vi "main_real-time HMI for air-wrting to input characters 23.3.3.vi"() -> ()   [LabVIEW 2020]
uses:
  <vilib>/Analysis/3filter.llb/Filter Passband Type.ctl
  <vilib>/Analysis/NI_AALBase.lvlib
  <vilib>/Analysis/3filter.llb/Butterworth Filter (DBL).vi
  <vilib>/express/express analysis/Spectral/XNode/ExpressSpectralMeasurementsBlockNode.xnode
  <vilib>/express/express analysis/Spectral/Block/exnSpectralBlock spectral measurements power poly.vi
  <vilib>/Analysis/NI_AALPro.lvlib
  <vilib>/Analysis/NI_AAL_SigProc.lvlib
  <vilib>/Utility/file.llb/Write Delimited Spreadsheet (DBL).vi
  <vilib>/express/express analysis/Spectral/Block/exnSpectralBlock spectral measurements power DDT.vi
panel:
  out "最大值 2":dbl
  out "手势":dbl
  in  "训练——手势":string
  out "卡尔曼滤波":cluster{"Y":dbl[], "Y":dbl[]}[](graph)
  out "通道1":dynamicdata(graph)
  out "XY Graph 2":cluster{"Y":dbl[], "Y":dbl[]}[](graph) caption="ML_集成树"
  in  "训练——位置":dbl
  out "数值":dbl
  out "采样点 2":dbl
  out "采样点":dbl
  out "ToF 2(cm)":dbl
  out "ToF 1(cm)":dbl
  out "有手势":bool
  out "最大值 1":dbl
  out "最大值2":dbl
  out "波形图 2":dbl[](graph)
  out "余数 2":dbl
  out "循环 2":dbl
  out "波形图":dbl[](graph)
  out "通道1_去环境噪声":dbl[](graph)
  out "通道2_去环境+滤波":dbl[](graph)
  out "频谱2":dynamicdata(graph)
  out "通道1_滤波":dbl[](graph)
  out "通道2_滤波":dbl[](graph)
  out "激励信号":dynamicdata(graph)
  out "通道2":dynamicdata(graph)
  in  "停止":bool
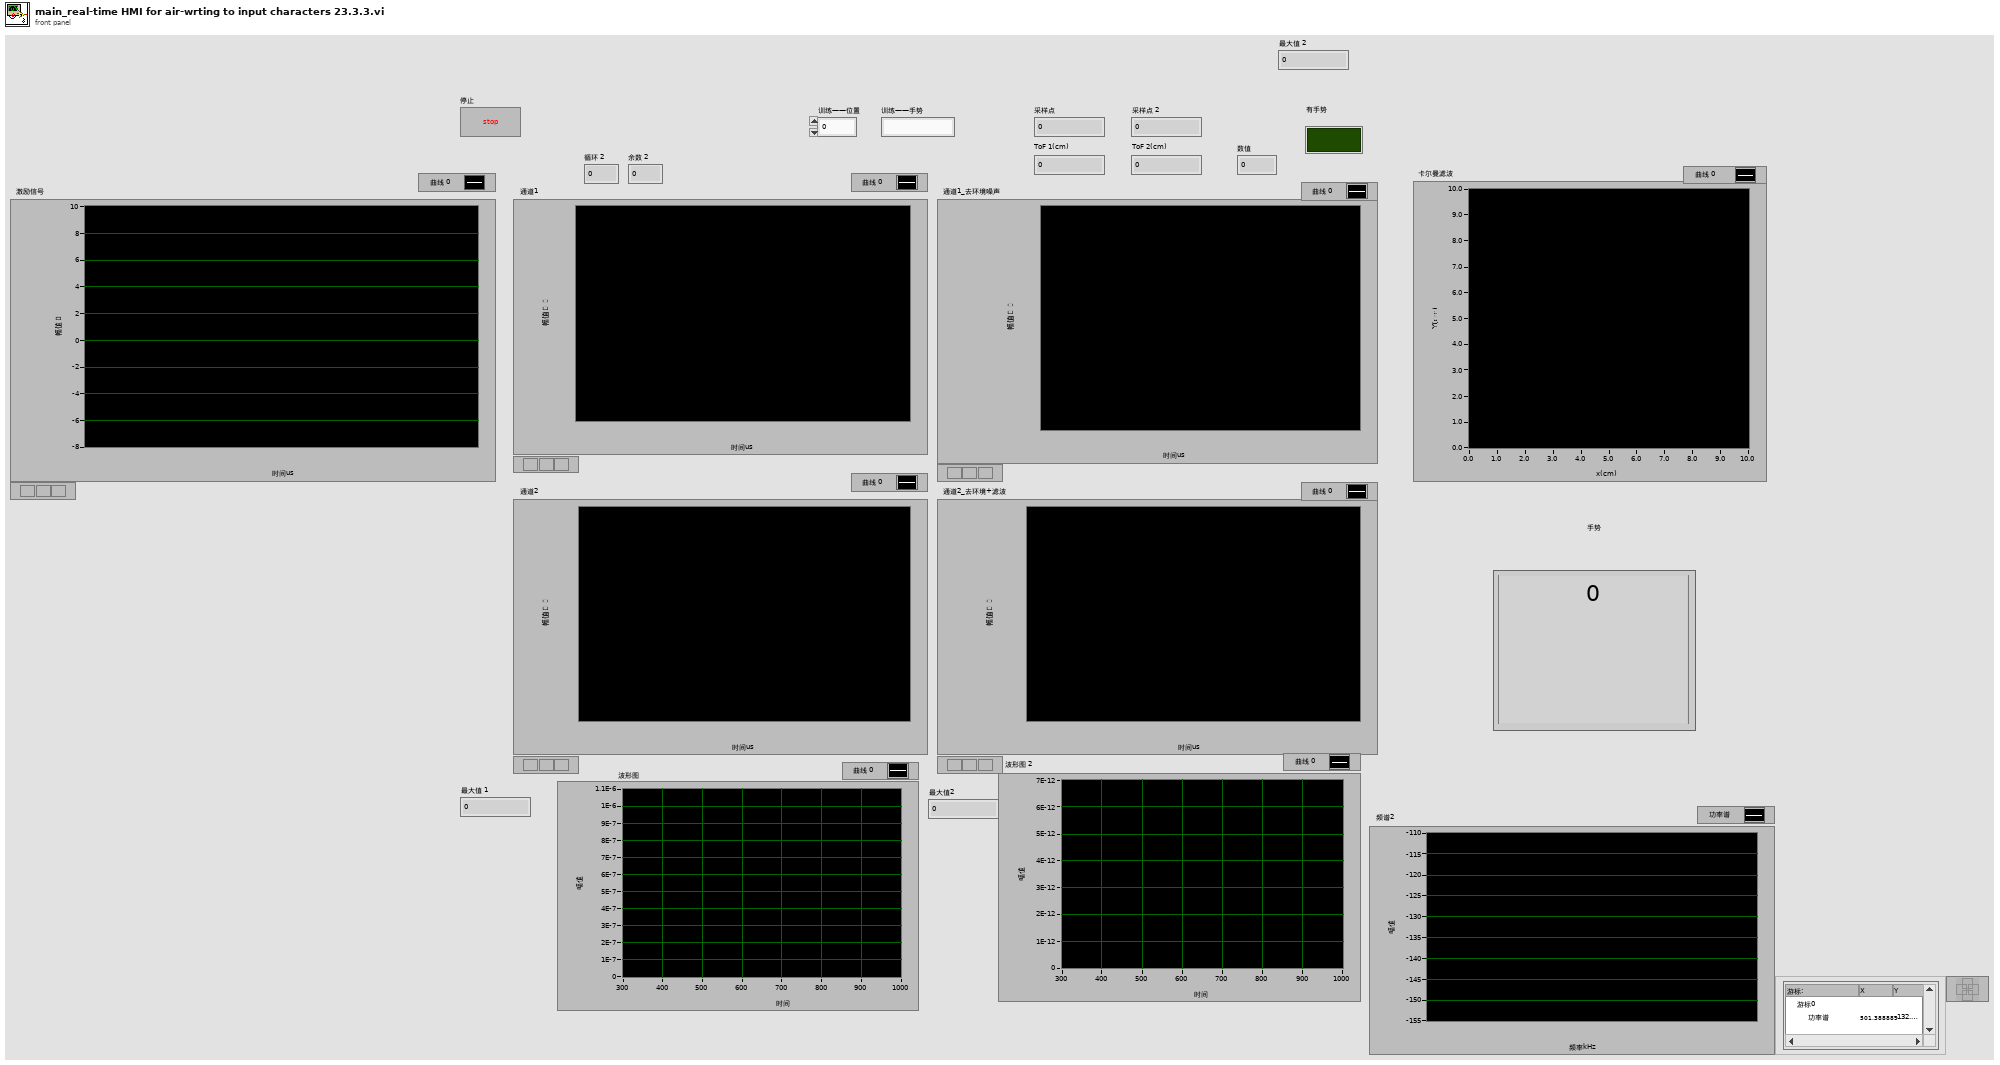
[diagram p1: front panel]
types:
  T1 = typedef "NI_AALBase.lvlib/Filter Passband Type.ctl" = enum32{"Lowpass", "Highpass", "Bandpass", "Bandstop"}
  T2 = cluster{"averaging mode":u16, "weighting mode":u16, "number of averages":u32}
  T3 = cluster{"dB On (F)":bool, "unwrap phase (F)":bool, "convert to degree (F)":bool}
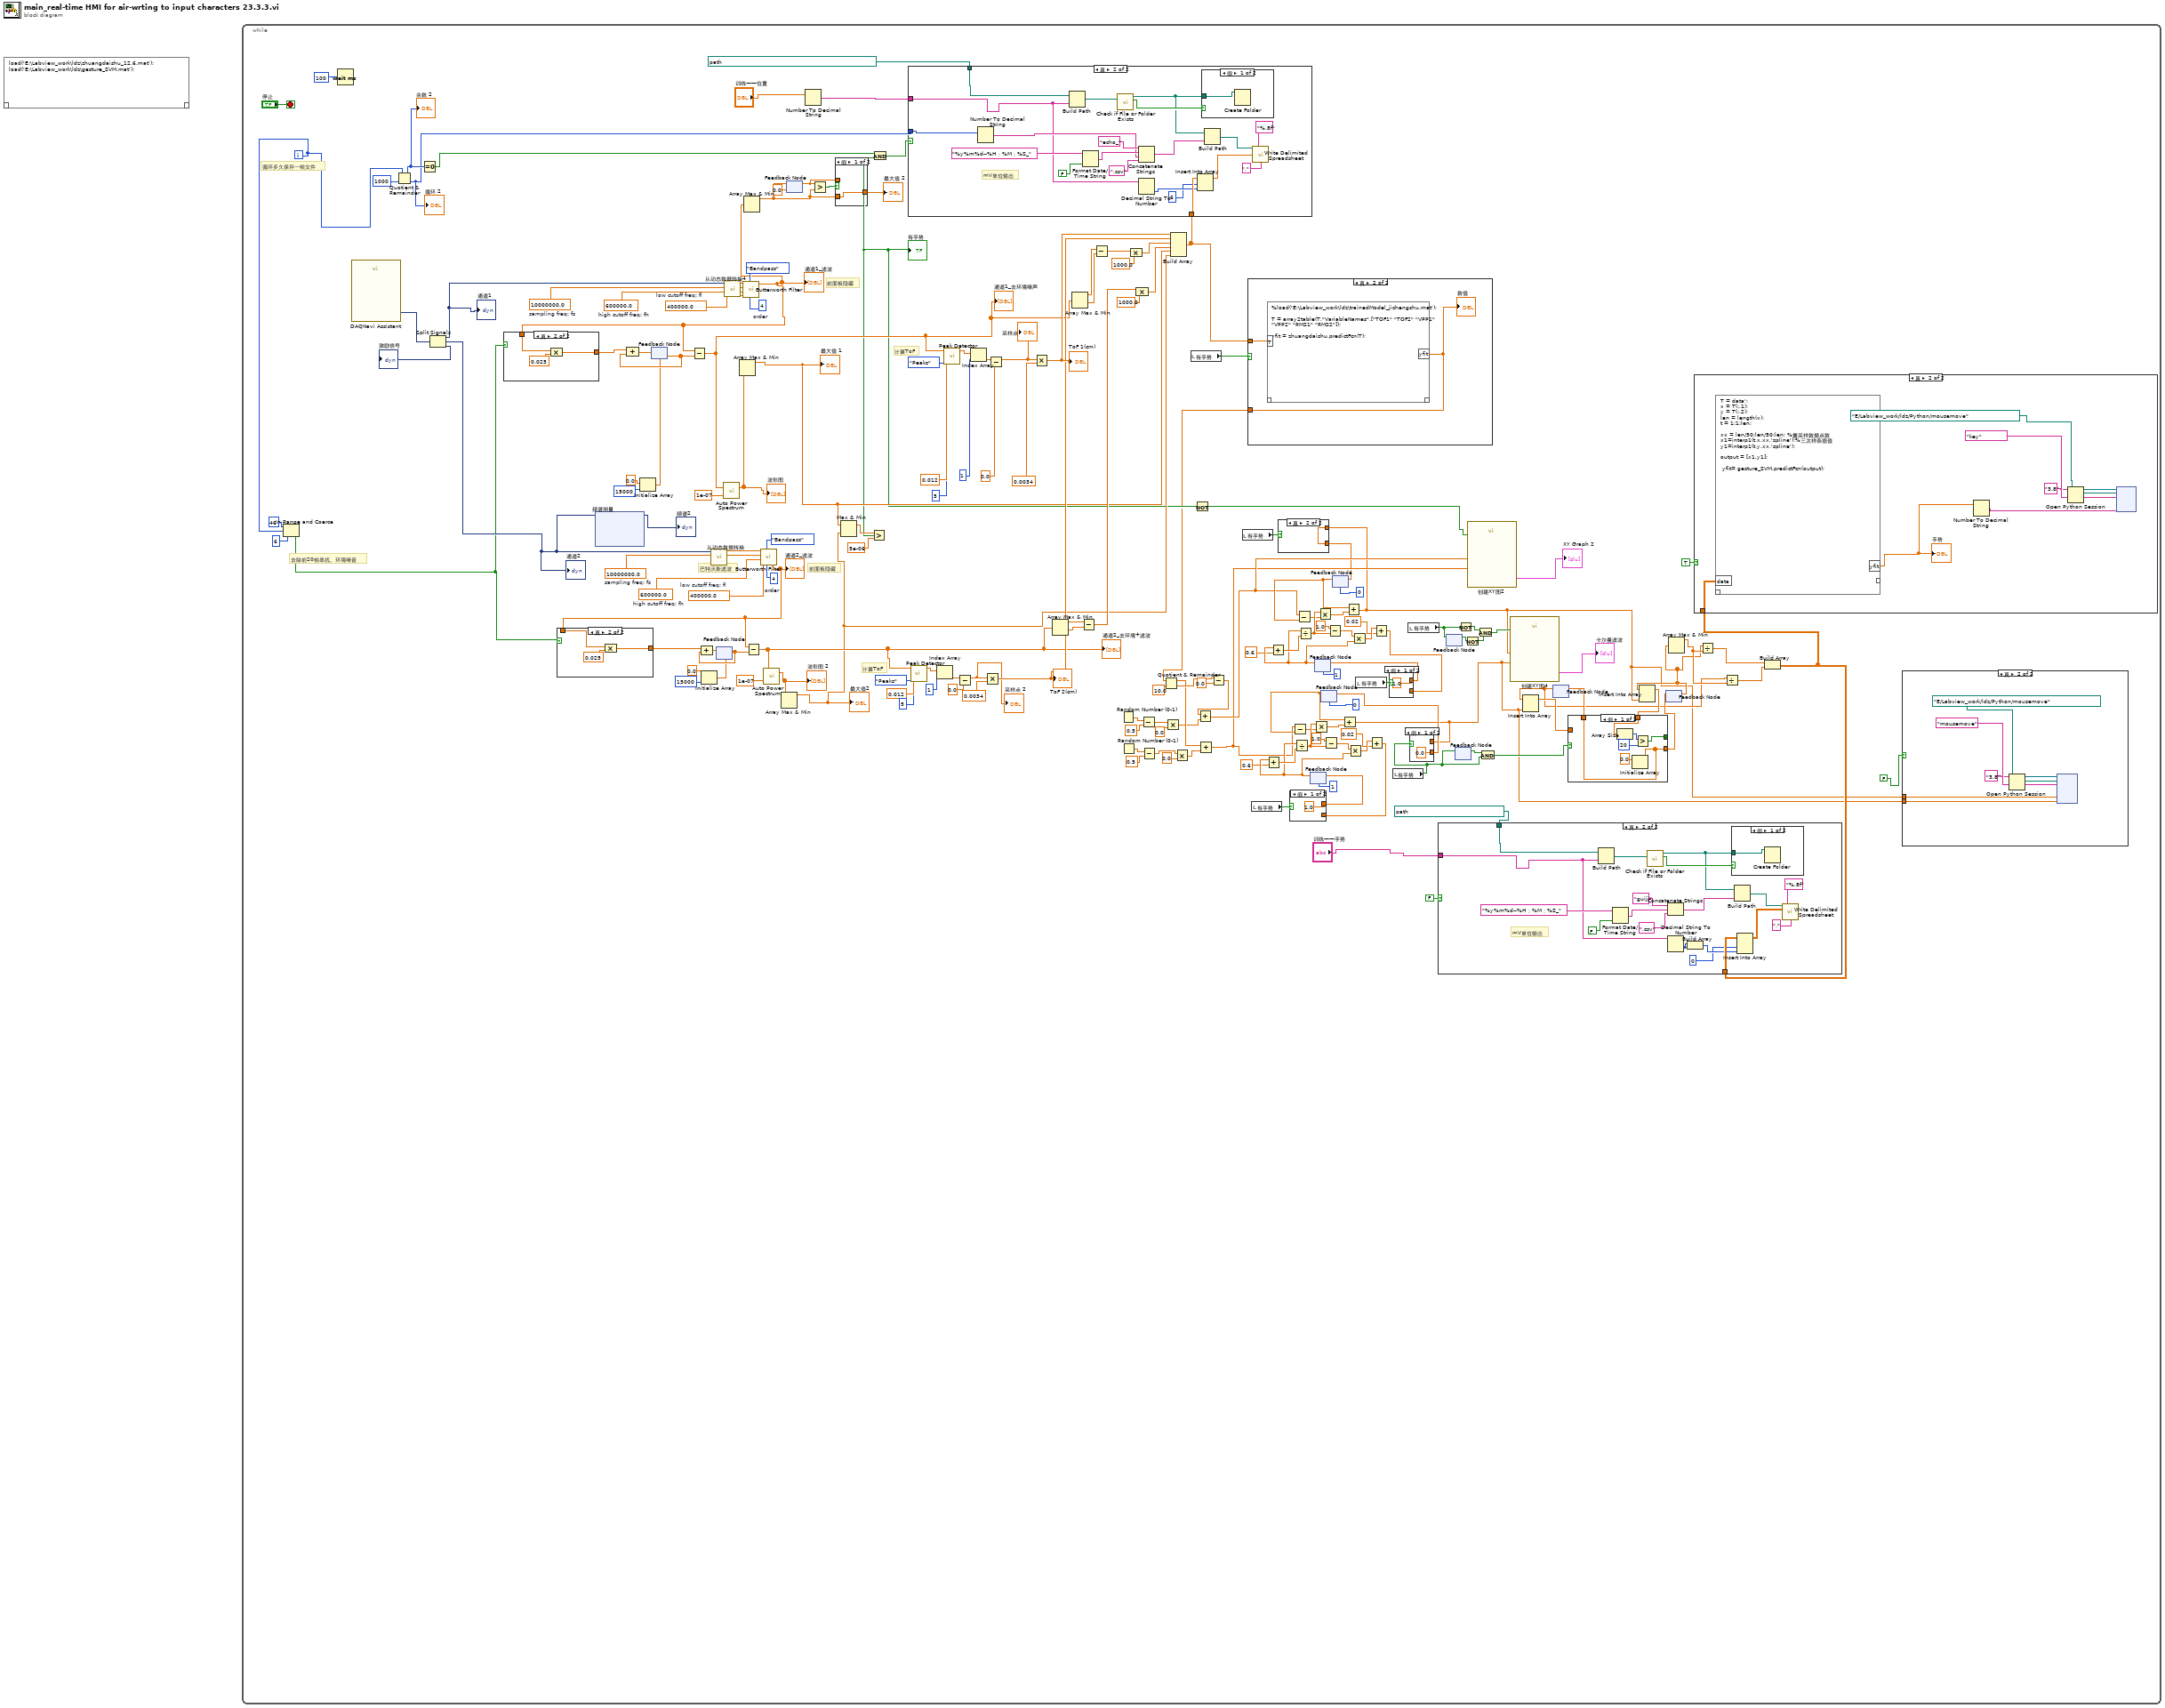
[diagram p0: block diagram]
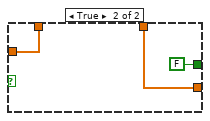
[diagram p7: hidden frame]
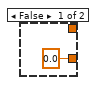
[diagram p11: hidden frame]
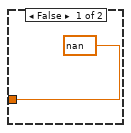
[diagram p12: hidden frame]
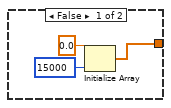
[diagram p15: hidden frame]
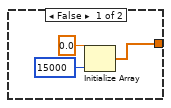
[diagram p16: hidden frame]
diagram:
  n1 = script code="load('E:\\Labview_work\\ldz\\zhuangdaishu_12.6.mat');\nload('E:\\Labview_work\\ldz\\gesture_SVM.mat');"() -> ()  [unwired: 1 in, 1 out]
  n2 = while {
    i -> [w139]
    stop <- "停止" stop-if-true
    w161 = 400000.0  # low cutoff freq: fl
    w165 = 600000.0  # high cutoff freq: fh
    w164 = 10000000.0  # sampling freq: fs
    w166 = 4  # order
    w172 = 400000.0  # low cutoff freq: fl
    w171 = 600000.0  # high cutoff freq: fh
    w170 = 10000000.0  # sampling freq: fs
    w173 = 4  # order
    # "计算ToF"
    # "计算ToF"
    # "前面板隐藏"
    # "前面板隐藏"
    # "去除前20帧串扰、环境噪音"
    # "循环多久保存一帧文件"
    # "巴特沃斯滤波"
    n3 = In Range and Coerce(upper limit=46 ("上限"), x=w139, lower limit=6 ("下限")) -> (In Range?=w143:bool)  [unwired: 1 out]
    n4 = Wait (ms)(milliseconds to wait=100) -> ()  [unwired: 1 out]
    n5 = call "DAQNavi Assistant"() -> ("data out(DDT)"=w159:dynamicdata)  [unwired: 6 in, 21 out]
    n6 = Quotient & Remainder(x=w139, y=1000) -> (x-y*floor(x/y)=w141:i32, floor(x/y)=w140:i32)
    "循环 2" <- w140
    "余数 2" <- w141
    n7 = Equal To 0?(x=w141) -> (x = 0?=w130:bool)
    n8 = Split Signals(w159) -> (w93:dynamicdata, w160:dynamicdata, →"激励信号":dynamicdata)  [unwired: 3 in]
    "通道2" <- w160
    "通道1" <- w93
    n9 = xnode "频谱测量"("信号"=w160) -> ("功率谱"=→"频谱2":dynamicdata)  [unwired: 1 in, 1 out]
    n10 = Initialize Array(0.0 ("元素"), 15000 ("维数大小")) -> (w147:dbl[])
    n11 = feedback #1(w147) -> (w149:dbl[])
    n12 = Initialize Array(0.0 ("元素"), 15000 ("维数大小")) -> (w155:dbl[])
    n13 = call "从动态数据转换"("Dynamic Data Type"=w160) -> ("Array"=w168:dbl[])  [unwired: 3 in]
    n14 = feedback #2(w155) -> (w156:dbl[])
    n15 = call "从动态数据转换4"("Dynamic Data Type"=w93) -> ("Array"=w162:dbl[])  [unwired: 3 in]
    n16 = call-poly <vilib>:"Butterworth Filter.vi"("order"=w166, "filter type"=Filter_Passband_Type."Bandpass", "low cutoff freq: fl"=w161, "high cutoff freq: fh"=w165, "sampling freq: fs"=w164, "X"=w162) -> ("Filtered X"=w6:dbl[])  [unwired: 2 in, 1 out]
    "通道1_滤波" <- w6
    n17 = case shown="真" w143 {
      tunnel: w6 -> [_ w254]
      tunnel: [w251 w256] -> w151
      frame False {
        n18 = Initialize Array(0.0 ("元素"), 15000 ("维数大小")) -> (w251:dbl[])
      }
      frame True {
        n19 = Compound Arithmetic op=MULTIPLY(w254, 0.025) -> (w256:dbl[])
      }
    }
    n20 = Compound Arithmetic op=ADD(w151, w149) -> (w150:dbl[])
    n21 = feedback-in #1(w150) -> ()
    n22 = Subtract(x=w6, y=w149) -> (x-y=w109:dbl[])
    "通道1_去环境噪声" <- w109
    n23 = call <vilib>:"Auto Power Spectrum.vi"("dt"=1e-07, "Signal (V)"=w109) -> ("Power Spectrum (V^2 rms)"=w133:dbl[])  [unwired: 1 out]
    "波形图" <- w133
    n24 = Array Max & Min(array=w133) -> (max value=w100:dbl)  [unwired: 3 out]
    "最大值 1" <- w100
    n25 = Array Max & Min(array=w6) -> (max value=w3:dbl)  [unwired: 3 out]
    n26 = call-poly <vilib>:"Butterworth Filter.vi"("order"=w173, "filter type"=Filter_Passband_Type."Bandpass", "low cutoff freq: fl"=w172, "high cutoff freq: fh"=w171, "sampling freq: fs"=w170, "X"=w168) -> ("Filtered X"=w152:dbl[])  [unwired: 2 in, 1 out]
    "通道2_滤波" <- w152
    n27 = case shown="真" w143 {
      tunnel: w152 -> [_ w262]
      tunnel: [w257 w261] -> w158
      frame False {
        n28 = Initialize Array(0.0 ("元素"), 15000 ("维数大小")) -> (w257:dbl[])
      }
      frame True {
        n29 = Compound Arithmetic op=MULTIPLY(w262, 0.025) -> (w261:dbl[])
      }
    }
    n30 = Compound Arithmetic op=ADD(w158, w156) -> (w157:dbl[])
    n31 = feedback-in #2(w157) -> ()
    n32 = Subtract(x=w152, y=w156) -> (x-y=w108:dbl[])
    "通道2_去环境+滤波" <- w108
    n33 = call <vilib>:"Auto Power Spectrum.vi"("dt"=1e-07, "Signal (V)"=w108) -> ("Power Spectrum (V^2 rms)"=w134:dbl[])  [unwired: 1 out]
    "波形图 2" <- w134
    n34 = Array Max & Min(array=w134) -> (max value=w99:dbl)  [unwired: 3 out]
    "最大值2" <- w99
    n35 = feedback #3(0.0) -> (w2:dbl)
    n36 = feedback-in #3(w3) -> ()
    n37 = Number To Decimal String(number="训练——位置") -> (decimal integer string=w95:string)  [unwired: 1 in]
    n38 = Greater?(x=w2, y=w3) -> (0:w4:bool)
    n39 = case shown="假" w4 {
      tunnel: w3 -> [w175 _]
      tunnel: w2 -> [_ w176]
      tunnel: [w175 w176] -> w1
      frame False {
      }
      frame True {
      }
    }
    "最大值 2" <- w1
    n40 = Max & Min(x=w100, y=w99) -> (max(x,y)=w132:dbl)  [unwired: 1 out]
    n41 = Greater?(x=w132, y=5e-06) -> (0:w98:bool)
    "有手势" <- w98
    n42 = And(x=w130, y=w98) -> (x .and. y?=w129:bool)
    n43 = call <vilib>:"Peak Detector.vi"("peaks/valleys"=enum32{"Peaks", "Valleys"}."Peaks", "width"=5, "threshold"=0.012, "X"=w108) -> ("Locations"=w120:dbl[])  [unwired: 3 in, 4 out]
    n44 = Index Array(array=w120, index=1 ("索引")) -> (element=w89:dbl)
    n45 = call <vilib>:"Peak Detector.vi"("peaks/valleys"=enum32{"Peaks", "Valleys"}."Peaks", "width"=5, "threshold"=0.012, "X"=w109) -> ("Locations"=w125:dbl[])  [unwired: 3 in, 4 out]
    n46 = Subtract(x=w89, y=0.0) -> (x-y=w90:dbl)
    "采样点 2" <- w90
    n47 = Index Array(array=w125, index=1 ("索引")) -> (element=w118:dbl)
    n48 = Multiply(x=w90, y=0.0034) -> (x*y=w113:dbl)
    "ToF 2(cm)" <- w113
    n49 = Subtract(x=w118, y=0.0) -> (x-y=w92:dbl)
    "采样点" <- w92
    n50 = Multiply(x=w92, y=0.0034) -> (x*y=w114:dbl)
    "ToF 1(cm)" <- w114
    n51 = Array Max & Min(array=w108) -> (max value=w103:dbl, min value=w102:dbl)  [unwired: 2 out]
    n52 = Array Max & Min(array=w109) -> (max value=w107:dbl, min value=w106:dbl)  [unwired: 2 out]
    n53 = Subtract(x=w103, y=w102) -> (x-y=w104:dbl)
    n54 = Subtract(x=w107, y=w106) -> (x-y=w105:dbl)
    n55 = Random Number (0-1)() -> (number: 0 to 1=w84:dbl)
    n56 = Random Number (0-1)() -> (number: 0 to 1=w81:dbl)
    n57 = Compound Arithmetic op=MULTIPLY(w105, 1000.0) -> (w111:dbl)
    n58 = Compound Arithmetic op=MULTIPLY(w104, 1000.0) -> (w101:dbl)
    n59 = Subtract(x=w84, y=0.5) -> (x-y=w78:dbl)
    n60 = Subtract(x=w81, y=0.5) -> (x-y=w73:dbl)
    n61 = Multiply(x=w78, y=0.0) -> (x*y=w77:dbl)
    n62 = Build Array(w114, w113, w111, w101, w100, w99) -> (w97:dbl[])
    n63 = case shown="真" w129 {
      tunnel: w140 -> [_ w240]
      tunnel: path "E:/Labview_work/ldz/数据/3.3/test" ("路径") -> [_ w237]
      tunnel: w97 -> [_ w235]
      tunnel: w95 -> [_ w230]
      frame False {
      }
      frame True {
        # "mV单位输出"
        n64 = Number To Decimal String(number=w240) -> (decimal integer string=w239:string)  [unwired: 1 in]
        n65 = Build Path(base path=w237, name or relative path=w230) -> (appended path=w244:path)
        n66 = Format Date/Time String ("格式化日期/时间字符串")(time format string (%c)="%y%m%d--%H：%M：%S_", UTC format=FALSE) -> (date/time string=w246:string)  [unwired: 1 in]
        n67 = call <vilib>:"Check if File or Folder Exists.vi"("path"=w244) -> ("file or folder exists?"=w243:bool, "dup path"=w231:path)  [unwired: 8 in, 1 out]
        n68 = Concatenate Strings("echo_" ("字符串"), w246, w239, ".csv" ("字符串")) -> (w248:string)
        n69 = Decimal String To Number(string=w230) -> (number=w233:i32)  [unwired: 2 in, 1 out]
        n70 = Insert Into Array(array=w235, index=6 ("索引"), new element=w233) -> (w234:dbl[])
        n71 = case shown="假" w243 {
          tunnel: w231 -> [w250 _]
          frame False {
            n72 = Create Folder(path (use dialog)=w250) -> ()  [unwired: 2 in, 3 out]
          }
          frame True {
          }
        }
        n73 = Build Path(base path=w231, name or relative path=w248) -> (appended path=w247:path)
        n74 = call-poly <vilib>:"Write Delimited Spreadsheet.vi"("file path (dialog if empty)"=w247, "format (%.3f)"="%.8f", "1D data"=w234, "delimiter (\\t)"="," ("delimiter (\\t)")) -> ()  [unwired: 10 in, 2 out]
      }
    }
    n75 = Multiply(x=w73, y=0.0) -> (x*y=w74:dbl)
    n76 = local read "有手势"() -> (w43:bool)
    n77 = Not(x=w98) -> (.not. x?=w28:bool)
    n78 = local read "有手势"() -> (w38:bool)
    n79 = case shown="真" w43 {
      tunnel: w97 -> [_ w229]
      tunnel: [nan w228] -> w46
      frame False {
      }
      frame True {
        n80 = script code="%load('E:\\Labview_work\\ldz\\trainedModel_jichengshu.mat');\n\nT = array2table(T,\"VariableNames\",[\"TOF1\" \"TOF2\" \"VPP1\" \"VPP2\" \"RMS1\" \"RMS2\"]);\n\nyfit = zhuangdaishu.predictFcn(T);" ("脚本节点")("T"=w229) -> ("yfit"=w228:dbl)  [unwired: 1 in, 1 out]
        "数值" <- w228
      }
    }
    n81 = Quotient & Remainder(x=w46, y=10.0) -> (x-y*floor(x/y)=w79:dbl, floor(x/y)=w86:dbl)
    n82 = Add(x=w79, y=w74) -> (x+y=w44:dbl)
    n83 = Subtract(x=w86, y=0.0) -> (x-y=w82:dbl)
    n84 = Add(x=w82, y=w77) -> (x+y=w45:dbl)
    n85 = local read "有手势"() -> (w36:bool)
    n86 = feedback #4(1) -> (w52:dbl)
    n87 = Add(x=w52, y=0.6) -> (x+y=w59:dbl)
    n88 = Divide(x=w52, y=w59) -> (x/y=w57:dbl)
    n89 = feedback #5(1) -> (w65:dbl)
    n90 = Add(x=w65, y=0.6) -> (x+y=w72:dbl)
    n91 = Divide(x=w65, y=w72) -> (x/y=w70:dbl)
    n92 = feedback #6(0) -> (w51:dbl)
    n93 = Subtract(x=w44, y=w51) -> (x-y=w56:dbl)
    n94 = Multiply(x=w57, y=w56) -> (x*y=w55:dbl)
    n95 = Subtract(x=1.0, y=w57) -> (x-y=w54:dbl)
    n96 = Subtract(x=1.0, y=w70) -> (x-y=w67:dbl)
    n97 = feedback #7(0) -> (w64:dbl)
    n98 = Subtract(x=w45, y=w64) -> (x-y=w69:dbl)
    n99 = Multiply(x=w70, y=w69) -> (x*y=w68:dbl)
    n100 = Add(x=w51, y=w55) -> (x+y=w11:dbl)
    n101 = Add(x=w64, y=w68) -> (x+y=w12:dbl)
    n102 = case shown="真" w38 {
      tunnel: w12 -> [_ w226]
      tunnel: [0.0 w226] -> w37
      frame False {
      }
      frame True {
      }
    }
    n103 = feedback-in #7(w37) -> ()
    n104 = Multiply(x=w54, y=w52) -> (x*y=w53:dbl)
    n105 = Multiply(x=w67, y=w65) -> (x*y=w66:dbl)
    n106 = local read "有手势"() -> (w31:bool)
    n107 = Add(x=w53, y=0.02) -> (x+y=w35:dbl)
    n108 = case shown="假" w36 {
      tunnel: w35 -> [_ w224]
      tunnel: [1.0 w224] -> w34
      frame False {
      }
      frame True {
      }
    }
    n109 = feedback-in #4(w34) -> ()
    n110 = Add(x=w66, y=0.02) -> (x+y=w33:dbl)
    n111 = case shown="假" w31 {
      tunnel: w33 -> [_ w222]
      tunnel: [1.0 w222] -> w32
      frame False {
      }
      frame True {
      }
    }
    n112 = feedback-in #5(w32) -> ()
    n113 = local read "有手势"() -> (w10:bool)
    n114 = local read "有手势"() -> (w29:bool)
    n115 = case shown="假" w10 {
      tunnel: w11 -> [_ w220]
      tunnel: [0.0 w220] -> w30
      frame False {
      }
      frame True {
      }
    }
    n116 = feedback-in #6(w30) -> ()
    n117 = feedback-in #8(w29) -> ()
    n118 = feedback #8() -> (w40:bool)  [unwired: 1 in]
    n119 = feedback #9() -> (w14:bool)  [unwired: 1 in]
    n120 = feedback-in #9(w10) -> ()
    n121 = Not(x=w29) -> (.not. x?=w42:bool)
    n122 = Not(x=w40) -> (.not. x?=w39:bool)
    n123 = call "创建XY图2"("Reset"=w28, "Y Input"=w44, "X Input"=w45) -> ("XY Graph"=→"XY Graph 2":cluster{"X":dbl[], "Y":dbl[]}[])  [unwired: 7 in, 1 out]
    n124 = And(x=w42, y=w39) -> (x .and. y?=w41:bool)
    n125 = And(x=w14, y=w10) -> (x .and. y?=w13:bool)
    n126 = call "创建XY图4"("Reset"=w41, "Y Input"=w11, "X Input"=w12) -> ("XY Graph"=→"卡尔曼滤波":cluster{"X":dbl[], "Y":dbl[]}[])  [unwired: 7 in, 1 out]
    n127 = feedback #10() -> (w18:dbl[])  [unwired: 1 in]
    n128 = Insert Into Array(array=w18, new element=w11) -> (w23:dbl[])  [unwired: 1 in]
    n129 = feedback #11() -> (w19:dbl[])  [unwired: 1 in]
    n130 = Insert Into Array(array=w19, new element=w12) -> (w24:dbl[])  [unwired: 1 in]
    n131 = case shown="假" w13 {
      tunnel: w24 -> [w214 w218]
      tunnel: [w210 w218] -> w20
      tunnel: [w211 FALSE] -> _
      tunnel: w23 -> [_ w216]
      tunnel: [w210 w216] -> w21
      frame False {
        n132 = Array Size(array=w214) -> (size(s)=w213:i32)
        n133 = Initialize Array(0.0 ("元素")) -> (w210:dbl[])  [unwired: 1 in]
        n134 = Greater?(x=w213, y=20) -> (0:w211:bool)
      }
      frame True {
      }
    }
    n135 = feedback-in #10(w21) -> ()
    n136 = feedback-in #11(w20) -> ()
    n137 = Array Max & Min(array=w19) -> (max value=w22:dbl)  [unwired: 3 out]
    n138 = Divide(x=w19, y=w22) -> (x/y=w17:dbl[])
    n139 = Divide(x=w18, y=w22) -> (x/y=w16:dbl[])
    n140 = Build Array(w17, w16) -> (w15:dbl[][])
    n141 = case shown="真" FALSE {
      tunnel: path "E:/Labview_work/ldz/数据/3.3/手势" ("路径") -> [_ w199]
      tunnel: "训练——手势" -> [_ w196]
      tunnel: w15 -> [_ w194]
      frame False {
      }
      frame True {
        # "mV单位输出"
        n142 = Build Path(base path=w199, name or relative path=w196) -> (appended path=w203:path)
        n143 = Format Date/Time String ("格式化日期/时间字符串")(time format string (%c)="%y%m%d--%H：%M：%S_", UTC format=FALSE) -> (date/time string=w205:string)  [unwired: 1 in]
        n144 = call <vilib>:"Check if File or Folder Exists.vi"("path"=w203) -> ("file or folder exists?"=w202:bool, "dup path"=w197:path)  [unwired: 8 in, 1 out]
        n145 = Concatenate Strings("guiji" ("字符串"), w205, ".csv" ("字符串")) -> (w207:string)
        n146 = Decimal String To Number(string=w196) -> (number=w193:i32)  [unwired: 2 in, 1 out]
        n147 = Build Array(w193, w193) -> (w192:i32[])
        n148 = case shown="假" w202 {
          tunnel: w197 -> [w209 _]
          frame False {
            n149 = Create Folder(path (use dialog)=w209) -> ()  [unwired: 2 in, 3 out]
          }
          frame True {
          }
        }
        n150 = Build Path(base path=w197, name or relative path=w207) -> (appended path=w206:path)
        n151 = Insert Into Array(array=w194, index (col)=0 ("索引"), new element=w192) -> (w190:dbl[][])  [unwired: 1 in]
        n152 = call-poly <vilib>:"Write Delimited Spreadsheet.vi"("file path (dialog if empty)"=w206, "format (%.3f)"="%.8f", "2D data"=w190, "delimiter (\\t)"="," ("delimiter (\\t)")) -> ()  [unwired: 10 in, 2 out]
      }
    }
    n153 = case shown="真" TRUE {
      tunnel: w15 -> [_ w189]
      frame False {
      }
      frame True {
        n154 = script code="T = data';\nx = T(:,1);\ny = T(:,2);\nlen = length(x);\nt = 1:1:len;\n\nxx = len/50:len/50:len; %重采样数据点数\nx1=interp1(t,x,xx,'spline');%三次样条插值\ny1=interp1(t,y,xx,'spline');\n\noutput = [x1,y1];\n\n yfit= gesture_SVM.predictFcn(output);"("data"=w189) -> ("yfit"=w184:dbl)  [unwired: 1 in, 1 out]
        "手势" <- w184
        n155 = Number To Decimal String(number=w184) -> (decimal integer string=w183:string)  [unwired: 1 in]
        n156 = Open Python Session(python version="3.8" ("Python版本")) -> (session out=w185:refnum<k35>)  [unwired: 2 in, 1 out]
        n157 = node(w185, path "E:/Labview_work/ldz/Python/mousemove" ("路径"), "key" ("字符串"), w183) -> ()  [unwired: 4 in, 4 out]
      }
    }
    n158 = case shown="真" FALSE {
      tunnel: w12 -> [_ w178]
      tunnel: w11 -> [_ w177]
      frame False {
      }
      frame True {
        n159 = Open Python Session(python version="3.8" ("Python版本")) -> (session out=w179:refnum<k35>)  [unwired: 2 in, 1 out]
        n160 = node(w179, path "E:/Labview_work/ldz/Python/mousemove" ("路径"), "mousemove" ("字符串"), w178, w177) -> ()  [unwired: 5 in, 4 out]
      }
    }
  }
